vi "Open.vi"(8 "error in (no error)":errorcluster) -> (0 "error out":errorcluster)   [LabVIEW 2019]
uses:
  <vilib>/Utility/error.llb/Error Cluster From Error Code.vi
  <vilib>/ErrorRing/Error Ring.xnode
  Kernel32.dll
  source/repos/Kinova Labview Interface/Debug/KLInterface.dll
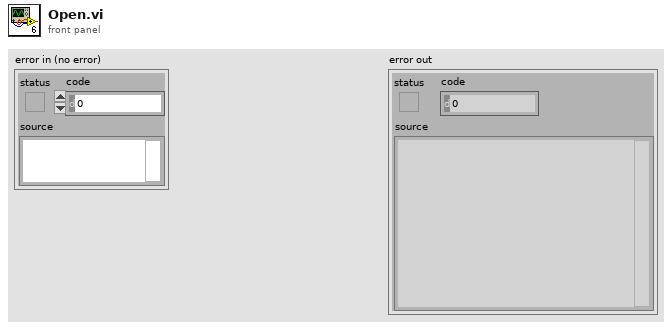
[diagram p1: front panel]
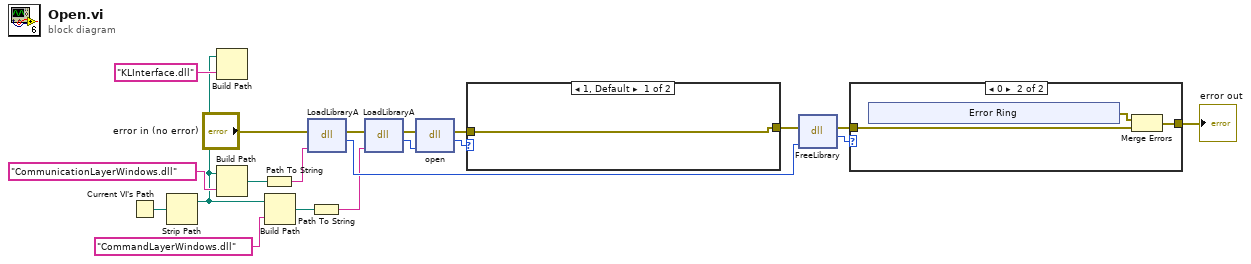
[diagram p0: block diagram]
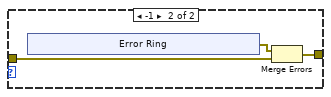
[diagram p3: hidden frame]
diagram:
  n1 = Current VI's Path() -> (path=w11:path)
  n2 = Strip Path(path=w11) -> (stripped path=w5:path)  [unwired: 1 out]
  n3 = Build Path(base path=w5, name or relative path="KLInterface.dll") -> ()  [unwired: 1 out]
  n4 = Build Path(base path=w5, name or relative path="CommunicationLayerWindows.dll") -> (appended path=w15:path)
  n5 = Path To String(path=w15) -> (string=w17:string)
  n6 = Build Path(base path=w5, name or relative path="CommandLayerWindows.dll") -> (appended path=w6:path)
  n7 = dll-call lib="Kernel32.dll" fn="LoadLibraryA"(error in="error in (no error)", "file"=w17) -> (error out=w2:errorcluster, "return type"=w20:u32)  [unwired: 3 in, 1 out]
  n8 = Path To String(path=w6) -> (string=w4:string)
  n9 = dll-call lib="Kernel32.dll" fn="LoadLibraryA"(error in=w2, "file"=w4) -> (error out=w1:errorcluster, "return type"=w3:u32)  [unwired: 3 in, 1 out]
  n10 = dll-call lib="C:/Users/mcjssdcc/source/repos/Kinova Labview Interface/Debug/KLInterface.dll" fn="open"(error in=w1, "commandlayer_handle"=w3) -> (error out=w13:errorcluster, "return type"=w12:i32)  [unwired: 3 in, 1 out]
  n11 = case shown="1, Default" w12 {
    tunnel: [w21 w23] -> w19
    tunnel: w13 -> [w21 w22]
    frame 1, Default {
    }
    frame -1 {
      n12 = xnode "Error Ring"() -> ("error out"=w24:errorcluster)
      n13 = Merge Errors(w24, w22) -> (w23:errorcluster)
    }
  }
  n14 = dll-call lib="Kernel32.dll" fn="FreeLibrary"(error in=w19, "hmodule"=w20) -> (error out=w8:errorcluster, "return type"=w9:i32)  [unwired: 3 in, 1 out]
  n15 = case shown="0" w9 {
    tunnel: [w30 w32] -> w10
    tunnel: w8 -> [w30 w31]
    frame 1, Default {
    }
    frame 0 {
      n16 = xnode "Error Ring"() -> ("error out"=w33:errorcluster)
      n17 = Merge Errors(w33, w31) -> (w32:errorcluster)
    }
  }
  "error out" <- w10
